vi "VARIABLES_FALLOS.vi"(11 "all rows":string[][](array[string])) -> (0 "MAX RMS RUEDAS":dbl[][](array[numeric]), 1 "all rows 4":string[][](array[string]), 2 "TAGS":string[][](array[string]), 3 "TIMESTAMP":dbl[](array[numeric]), 5 "deleted portion 4":string, 6 "VELOCIDAD":dbl[](array[numeric]), 7 "TEMPER":dbl[](array[numeric]))   [LabVIEW 2015]
uses:
  <vilib>/Utility/file.llb/Write Delimited Spreadsheet (string).vi
panel:
  out "decimal integer string":string[](array[string])
  out "Array 9":string[][](array[string])
  out "sum":i32
  out "index of element 2":i32
  out "all rows 3":string[][](array[string])
  out "array ok":string[][](array[string])
  out "Array 8":i32[](array[numeric])
  out "Array 6":string[](array[string])
  out "Array 5":i32[](array[numeric])
  out "index of element":i32
  out "x/y":dbl
  out "Array 4":string[][](array[string])
  out "LIMITE":i32
  out "deleted portion 5":i32
  out "size(s) 2":i32[](array[numeric])
  out "output array":string[](array[string])
  out "Array 3":string[](array[string])
  out "array w/ subset deleted 2":string[](array[string])
  out "array1":string[](array[string])
  out "deleted portion 2":string
  out "Array 7":string[][](array[string])
  out "array w/ subset deleted":string[](array[string])
  out "Array 2":string[][](array[string])
  out "Array":string[][](array[string])
  out "VELOCIDAD":string[](array[string])
  out "TEMPER":string[](array[string])
  out "TIMESTAMP":string
  out "deleted portion 3":i32
  out "deleted portion":i32
  out "size(s)":i32[](array[numeric])
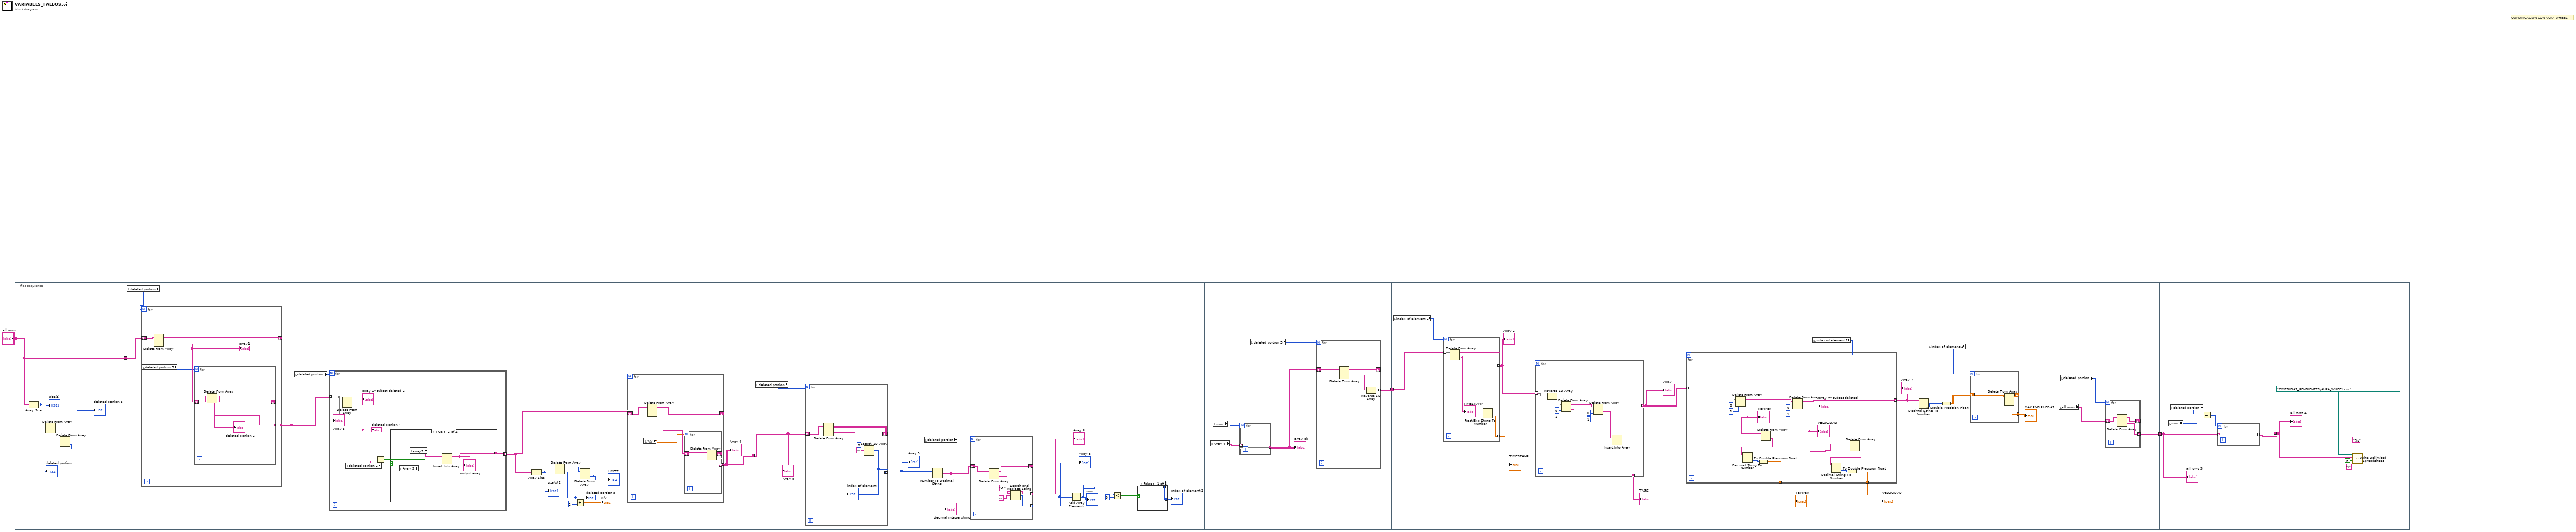
[diagram p0: block diagram]
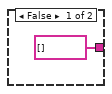
[diagram p2: hidden frame]
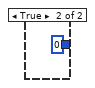
[diagram p3: hidden frame]
diagram:
  # "COMUNICACION CON AURA WHEEL"
  n1 = flat-sequence {
    tunnel: [w8] -> w7
    tunnel: "all rows" -> [w8]
    tunnel: w7 -> [w14]
    tunnel: [w13] -> w6
    tunnel: w6 -> [w32]
    tunnel: [w24] -> w2
    tunnel: w2 -> [w52]
    tunnel: [w81] -> w5
    tunnel: w5 -> [w101]
    tunnel: [w135] -> w4
    tunnel: w4 -> [w142]
    tunnel: [w141] -> w3
    tunnel: w3 -> [w151]
    frame #0 {
      n2 = Array Size(array=w8) -> (size(s)=w12:i32[])
      "size(s)" <- w12
      n3 = Delete From Array(array=w12) -> (deleted portion=→"deleted portion 3":i32, array with subset deleted=w11:i32[])  [unwired: 2 in]
      n4 = Delete From Array(array=w11) -> (deleted portion=→"deleted portion":i32)  [unwired: 2 in, 1 out]
    }
    frame #1 {
      n5 = local read "deleted portion"() -> (w15:i32)
      n6 = for {
        N: w15 -> [_]
        shift-right: [w19] -> _
        shift-left: w14 -> [w20]
        tunnel: [w16] -> w13 mode=indexing
        n7 = local read "deleted portion 3"() -> (w17:i32)
        n8 = Delete From Array(array=w20) -> (deleted portion=w18:string[], array with subset deleted=w19:string[][])  [unwired: 3 in]
        "array1" <- w18
        n9 = for {
          N: w17 -> [_]
          shift-right: [w22] -> _
          shift-left: w18 -> [w23]
          tunnel: [w21] -> w16 mode=indexing
          n10 = Delete From Array(array=w23) -> (deleted portion=w21:string, array with subset deleted=w22:string[])  [unwired: 2 in]
          "deleted portion 2" <- w21
        }
      }
    }
    frame #2 {
      n11 = local read "deleted portion"() -> (w33:i32)
      n12 = for {
        N: w33 -> [_]
        tunnel: w32 -> [w47] mode=indexing
        tunnel: [w42] -> w30 mode=indexing
        n13 = Delete From Array(array=w47) -> (deleted portion=w45:string, array with subset deleted=→"array w/ subset deleted 2":string[])  [unwired: 2 in]
        "deleted portion 4" <- w45
        n14 = local read "deleted portion 2"() -> (w44:string)
        n15 = Equal?(x=w45, y=w44) -> (x = y?=w43:bool)
        n16 = case shown="True" w43 {
          tunnel: [string[] [] ("array1") w49] -> w42
          frame False {
          }
          frame True {
            n17 = local read "Array 3"() -> (w50:string[])
            n18 = local read "array1"() -> (w51:string[])
            n19 = Insert Into Array(array=w51, new element=w50) -> (w49:string[])  [unwired: 1 in]
            "output array" <- w49
          }
        }
        "Array 3" <- w47
      }
      n20 = Array Size(array=w30) -> (size(s)=w31:i32[])
      "size(s) 2" <- w31
      n21 = Delete From Array(array=w31) -> (deleted portion=w27:i32, array with subset deleted=w29:i32[])  [unwired: 2 in]
      "deleted portion 5" <- w27
      n22 = Divide(x=w27, y=2) -> (x/y=→"x/y":dbl)
      n23 = Delete From Array(array=w29) -> (deleted portion=w28:i32)  [unwired: 2 in, 1 out]
      "LIMITE" <- w28
      n24 = for {
        N: w28 -> [_]
        shift-right: [w37] -> _
        shift-left: w30 -> [w38]
        tunnel: [w35] -> w24 mode=indexing
        n25 = local read "x/y"() -> (w34:dbl)
        n26 = Delete From Array(array=w38) -> (deleted portion=w36:string[], array with subset deleted=w37:string[][])  [unwired: 3 in]
        n27 = for {
          N: w34 -> [_]
          shift-right: [w40] -> _
          shift-left: w36 -> [w41]
          tunnel: [w39] -> w35 mode=indexing
          n28 = Delete From Array(array=w41) -> (deleted portion=w39:string, array with subset deleted=w40:string[])  [unwired: 2 in]
        }
      }
      "Array 4" <- w24
    }
    frame #3 {
      n29 = local read "deleted portion"() -> (w53:i32)
      n30 = for {
        N: w53 -> [_]
        shift-right: [w74] -> _
        shift-left: w52 -> [w73]
        tunnel: [w72] -> w55 mode=indexing
        n31 = Delete From Array(array=w73) -> (deleted portion=w77:string[], array with subset deleted=w74:string[][])  [unwired: 3 in]
        n32 = Search 1D Array(1D array=w77, element="", start index (0)=0) -> (index of element=w72:i32)
        "index of element" <- w72
      }
      "Array 5" <- w55
      n33 = local read "deleted portion"() -> (w54:i32)
      n34 = Number To Decimal String(number=w55) -> (decimal integer string=w56:string[])  [unwired: 1 in]
      "decimal integer string" <- w56
      n35 = for {
        N: w54 -> [_]
        shift-right: [w71] -> _
        shift-left: w56 -> [w70]
        tunnel: [w66] -> w57 mode=indexing
        tunnel: [w65] -> w61 mode=indexing
        n36 = Delete From Array(array=w70) -> (deleted portion=w69:string, array with subset deleted=w71:string[])  [unwired: 2 in]
        n37 = Search and Replace String(input string=w69, search string="-1", replace string="") -> (result string=w66:string, number of replacements=w65:i32)  [unwired: 5 in, 2 out]
      }
      "Array 6" <- w57
      "Array 8" <- w61
      n38 = Add Array Elements(numeric array=w61) -> (sum=w62:i32)
      "sum" <- w62
      n39 = Less?(x=w62, y=0) -> (x < y?=w59:bool)
      n40 = case shown="False" w59 {
        tunnel: [w63 0] -> w60
        tunnel: w62 -> [w63 _]
        frame False {
        }
        frame True {
        }
      }
      "index of element 2" <- w60
      "Array 9" <- w52
    }
    frame #4 {
      n41 = local read "Array 4"() -> (w80:string[][])
      n42 = local read "sum"() -> (w78:i32)
      n43 = for {
        N: w78 -> [_]
        tunnel: w80 -> [w83] mode=indexing
        tunnel: [w83] -> w79 mode=indexing
      }
      "array ok" <- w79
      n44 = local read "deleted portion 3"() -> (w82:i32)
      n45 = for {
        N: w82 -> [_]
        shift-right: [w86] -> _
        shift-left: w79 -> [w87]
        tunnel: [w84] -> w81 mode=indexing
        n46 = Delete From Array(array=w87) -> (deleted portion=w85:string[], array with subset deleted=w86:string[][])  [unwired: 3 in]
        n47 = Reverse 1D Array(array=w85) -> (reversed array=w84:string[])
      }
    }
    frame #5 {
      n48 = local read "index of element 2"() -> (w90:i32)
      n49 = for {
        N: w90 -> [_]
        tunnel: w101 -> [w134] mode=indexing
        tunnel: [w132] -> w100 mode=indexing
        tunnel: [w131] -> w95 mode=indexing
        n50 = Delete From Array(array=w134) -> (deleted portion=w133:string, array with subset deleted=w132:string[])  [unwired: 2 in]
        "TIMESTAMP" <- w133
        n51 = Fract/Exp String To Number(string=w133) -> (number=w131:dbl)  [unwired: 3 in, 1 out]
      }
      "Array 2" <- w100
      "TIMESTAMP" <- w95
      n52 = for {
        tunnel: w100 -> [w130] mode=indexing
        tunnel: [w123] -> w99 mode=indexing
        tunnel: [w120] -> w96 mode=indexing
        n53 = Reverse 1D Array(array=w130) -> (reversed array=w127:string[])
        n54 = Delete From Array(array=w127, length=1, index=0 ("index (row)")) -> (deleted portion=w121:string[], array with subset deleted=w124:string[])
        n55 = Delete From Array(array=w124, length=1, index=0 ("index (row)")) -> (deleted portion=w122:string[], array with subset deleted=w123:string[])
        n56 = Insert Into Array(array=w122, new element=w121) -> (w120:string[])  [unwired: 1 in]
      }
      "Array" <- w99
      "TAGS" <- w96
      n57 = local read "index of element 2"() -> (w89:i32)
      n58 = for {
        N: w89 -> [_]
        tunnel: w99 -> [w114] mode=indexing
        tunnel: [w107] -> w93 mode=indexing
        tunnel: [w106] -> w97 mode=indexing
        tunnel: [w105] -> w98 mode=indexing
        n59 = Delete From Array(array=w114, length=1, index=0 ("index (row)")) -> (deleted portion=w112:string[], array with subset deleted=w115:string[])
        "TEMPER" <- w112
        n60 = Delete From Array(array=w112) -> (deleted portion=w111:string)  [unwired: 2 in, 1 out]
        n61 = Decimal String To Number(string=w111) -> (number=w113:i32)  [unwired: 2 in, 1 out]
        n62 = To Double Precision Float(number=w113) -> (double precision float=w105:dbl)
        n63 = Delete From Array(array=w115, length=1, index=0 ("index (row)")) -> (deleted portion=w109:string[], array with subset deleted=w107:string[])
        "VELOCIDAD" <- w109
        "array w/ subset deleted" <- w107
        n64 = Delete From Array(array=w109) -> (deleted portion=w108:string)  [unwired: 2 in, 1 out]
        n65 = Decimal String To Number(string=w108) -> (number=w110:i32)  [unwired: 2 in, 1 out]
        n66 = To Double Precision Float(number=w110) -> (double precision float=w106:dbl)
      }
      "TEMPER" <- w98
      "VELOCIDAD" <- w97
      "Array 7" <- w93
      n67 = Decimal String To Number(string=w93) -> (number=w94:i32[][])  [unwired: 2 in, 1 out]
      n68 = local read "index of element 2"() -> (w88:i32)
      n69 = To Double Precision Float(number=w94) -> (double precision float=w92:dbl[][])
      n70 = for {
        N: w88 -> [_]
        shift-right: [w103] -> _
        shift-left: w92 -> [w104]
        tunnel: [w102] -> w91 mode=indexing
        n71 = Delete From Array(array=w104) -> (deleted portion=w102:dbl[], array with subset deleted=w103:dbl[][])  [unwired: 3 in]
      }
      "MAX RMS RUEDAS" <- w91
    }
    frame #6 {
      n72 = local read "all rows"() -> (w136:string[][])
      n73 = local read "deleted portion"() -> (w137:i32)
      n74 = for {
        N: w137 -> [_]
        shift-right: [w139] -> _
        shift-left: w136 -> [w140]
        tunnel: [w138] -> w135 mode=indexing
        n75 = Delete From Array(array=w140) -> (deleted portion=w138:string[], array with subset deleted=w139:string[][])  [unwired: 3 in]
      }
    }
    frame #7 {
      n76 = local read "sum"() -> (w145:i32)
      n77 = local read "deleted portion"() -> (w143:i32)
      n78 = Subtract(x=w143, y=w145) -> (x-y=w144:i32)
      n79 = for {
        N: w144 -> [_]
        tunnel: w142 -> [w146] mode=indexing
        tunnel: [w146] -> w141 mode=indexing
      }
      "all rows 3" <- w142
    }
    frame #8 {
      n80 = call-poly <vilib>:"Write Delimited Spreadsheet.vi"("file path (dialog if empty)"=path "C:/MEDIDAS_PENDIENTES/AURA_WHEEL.csv", "format (%s)"="%s", "2D data"=w151, "append to file? (F)"=FALSE, "delimiter (\\t)"=";" ("delimiter (\\t)")) -> ()  [unwired: 9 in, 2 out]
      "all rows 4" <- w151
    }
  }
